vi "UDS(queue).vi"() -> ()   [LabVIEW 2020]
uses:
  <vilib>/Automotive Diagnostic Command Set/Diagnostic Transport.llb/Transport Protocol Selector.ctl
  <vilib>/Automotive Diagnostic Command Set/Diagnostic Transport.llb/Property ID.ctl
  <vilib>/addons/Automotive Diagnostic Command Set/NI_Automotive Diagnostic Command Set.lvlib
panel:
  out "Clear DTC":bool
  in  "Auto":bool
  in  "Reset":bool
  in  "Stop":bool
  in  "Option":i32(ring) items=["读软件版本", "读DTC", "清DTC"]
  in  "Action":bool
  out "open_ok?":bool
  out "Response":u8[](array[numeric]) format="%.0x"
  out "CAN_log":string[][](table)
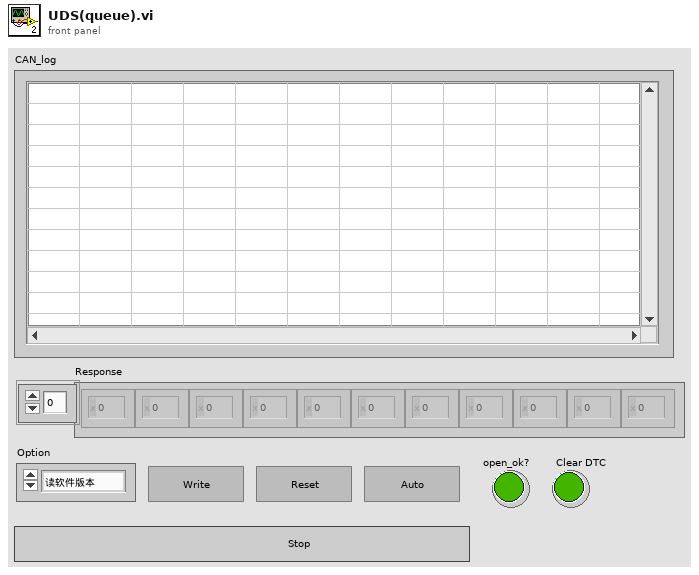
[diagram p1: front panel]
types:
  T1 = typedef "NI_Automotive Diagnostic Command Set.lvlib/Property ID.ctl" = enum16{"Timeout Diag Command", "Timeout FC (Bs)", "Timeout CF (Cr)", "Receive Block Size (BS)", "Wait Time CF (STmin)", "Max Wait Frames (N_WFTmax)", "Wait Frames to Send (N_WAIT)", "Time between Waits (T_W)", "Fill CAN Frames", "Fill Byte", "Invalid Response as Error", "Max RspPending Count", "VWTP Command Timeout", "STmin", "P2min", "Termination", "Timeout RspPending", "LIN Sleep", "Actual CAN IO Mode", "Response Plausibility Check", "Session-based Properties"}
  T2 = typedef "NI_Automotive Diagnostic Command Set.lvlib/Transport Protocol Selector.ctl" = enum16{"ISO TP - Normal Mode", "ISO TP - Mixed Mode", "VW TP 2.0", "Diagnostics on IP", "ISO TP LIN"}
  T3 = typedef "NI_Automotive Diagnostic Command Set.lvlib/Diag Reference.ctl" = cluster{"Diag CAN Handle":u32, "Transport Protocol":T2, "Receive Address Extension":u8, "Transmit Address Extension":u8, "Receive CAN Id":u32, "Transmit CAN Id":u32, "Log Frames ?":bool, "My TP Address":u8, "Other TP Address":u8, "T1":u16, "T2":u16, "T3":u16, "T4":u16, "Tx SN":u8, "Block Size":u8, "Rx SN":u8, "VW TP Initialized?":bool, "Tx block no":u8, "baud rate":u64, "Interface":string, "Channel Diag CAN Handle":u32, "UDP Connection ID":refnum<k16>, "TCP Connection ID":refnum<k5>, "Target IP Addr":u32, "Source Address":u16, "Target Address":u16, "Send Header NACK?":bool, "DLL Handle":u32, "NAD":u8, "Time Stamp read first":dbl, "Time Stamp read last":dbl, "Time Stamp write first":dbl, "Time Stamp write last":dbl, "Time Stamp write":dbl, "Time Stamp read":dbl, " I/O Mode":u32, "FD Baudrate":u64, "TX_DL":u16, "RX_DL":u16, "DoIP Protocol Version":T4, " Selected I/O Mode":u32, "TesterPresent Counter":u32, "TesterPresent Limit":u32, "TesterPresent Tick[ms]":i32, "TesterPresent RequireResponse?":bool, "TesterPresent Stored Ref?":bool, "TesterPresent Message":u8[], "TesterPresent Task Handle":i32, "TesterPresent Semaphore":T5, "Response Plausibility Check":u32, "Default Version?":bool, "Diagostic Globals":T6, "Session-based Properties?":bool}
  T4 = typedef "NI_Automotive Diagnostic Command Set.lvlib/DoIP Protocol Version.ctl" = u8
  T5 = typedef "Semaphore RefNum" = refnum<k1>
  T6 = typedef "NI_Automotive Diagnostic Command Set.lvlib/Diag Globals.ctl" = cluster{"Timeout FC (Bs)":u32, "Timeout CF (Cr)":u32, "Timeout Diag Command":u32, "Receive Block Size (BS)":u8, "Wait Time CF (STmin)":u8, "Max Waits (N_WFTmax)":u8, "Waits to Send (N_WAIT)":i32, "Time between Waits (TW)":u32, "Fill CAN Frames?":bool, "Fill Byte":u32, "Invalid Response as Error?":bool, "Max RspPending Count":u32, "VWTP Command Timeout":u32, "Transport Protocol":T2, "Diag CAN Handle":u32, "DLL Handle":u32, "Timeout RspPending":u32}
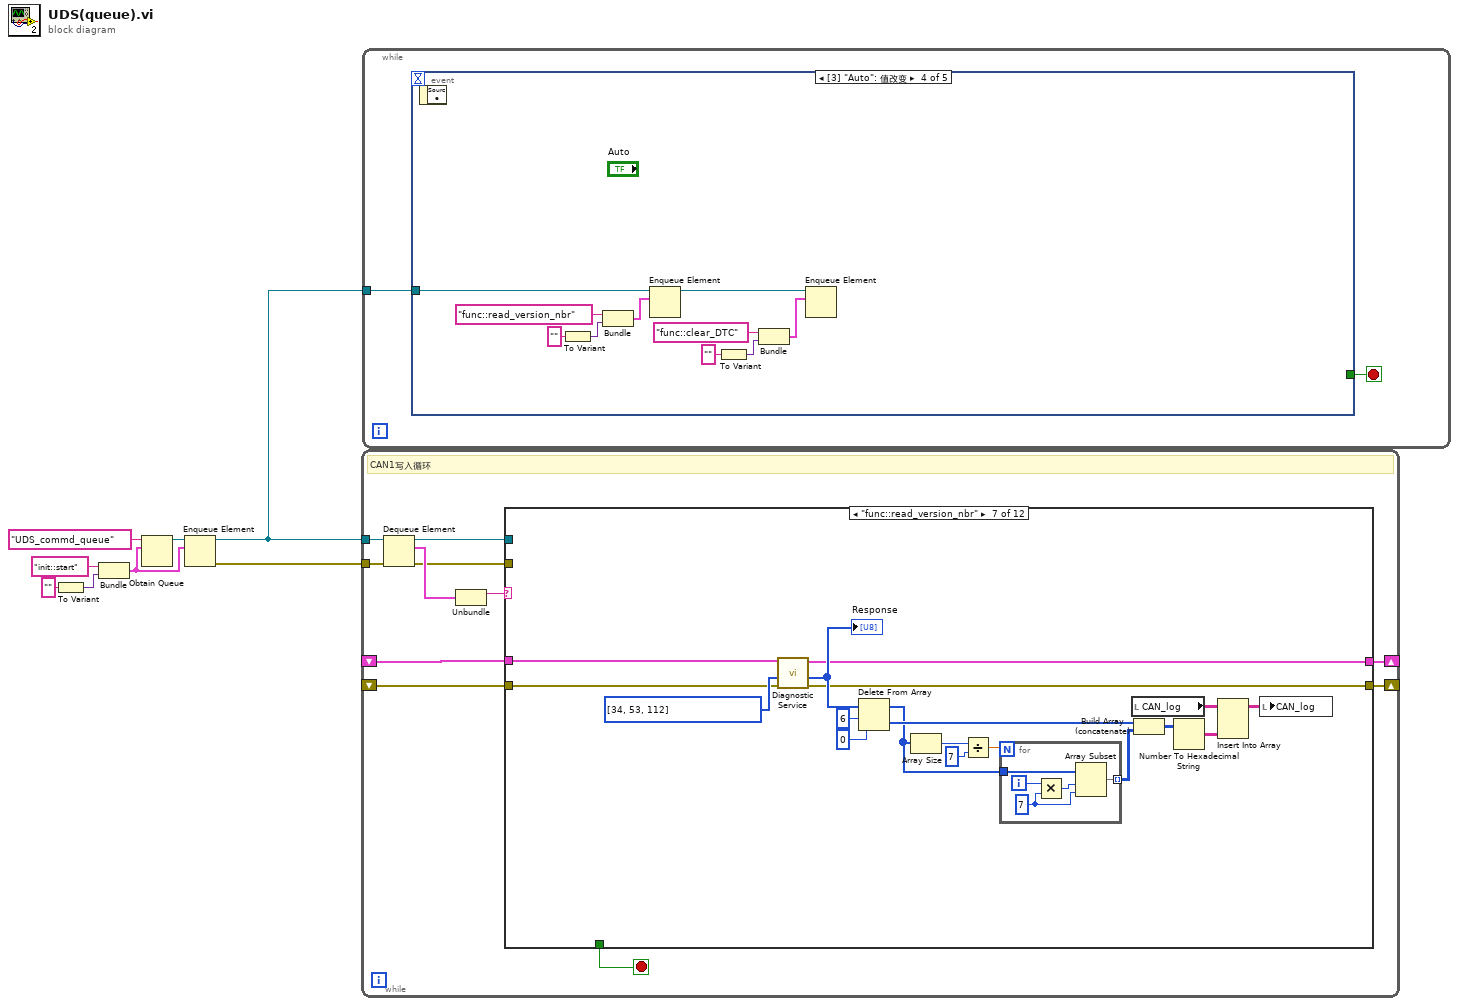
[diagram p0: block diagram]
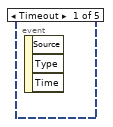
[diagram p2: hidden frame]
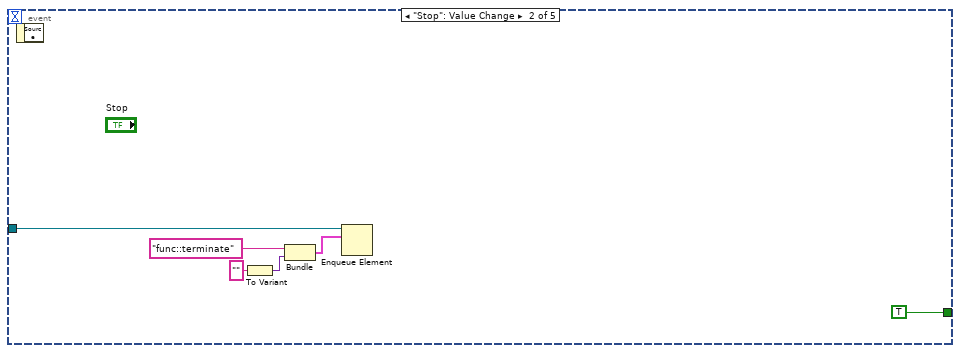
[diagram p3: hidden frame]
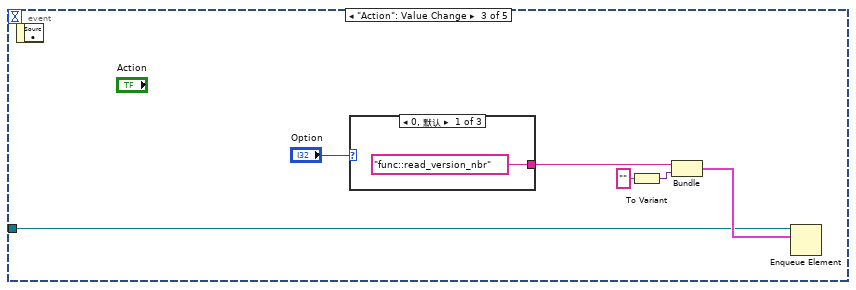
[diagram p4: hidden frame]
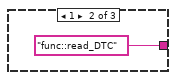
[diagram p5: hidden frame]
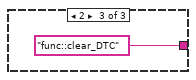
[diagram p6: hidden frame]
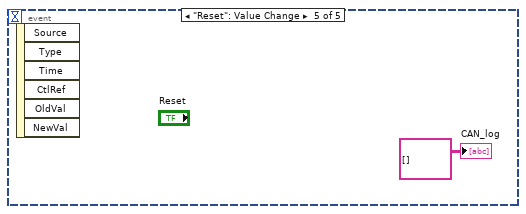
[diagram p7: hidden frame]
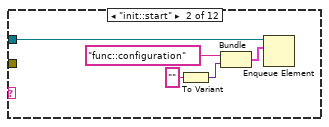
[diagram p9: hidden frame]
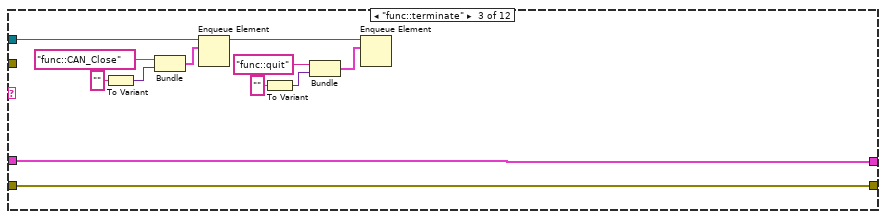
[diagram p10: hidden frame]
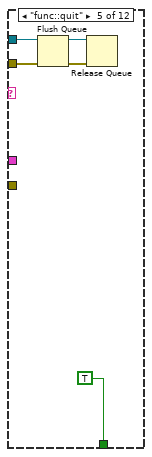
[diagram p12: hidden frame]
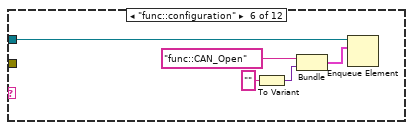
[diagram p13: hidden frame]
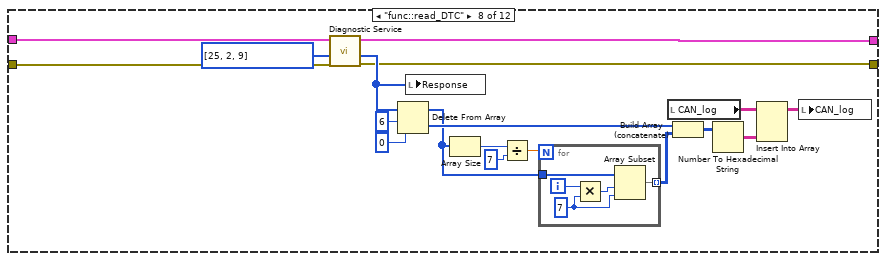
[diagram p14: hidden frame]
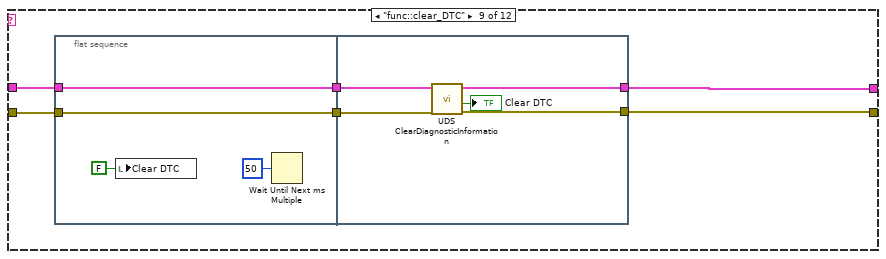
[diagram p15: hidden frame]
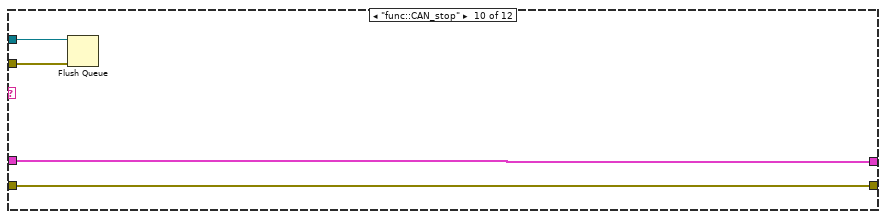
[diagram p16: hidden frame]
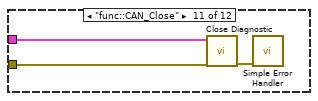
[diagram p17: hidden frame]
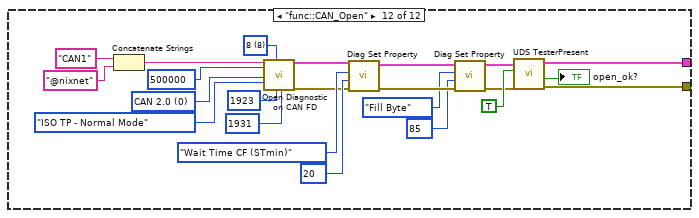
[diagram p18: hidden frame]
diagram:
  n1 = To Variant(anything="") -> (Variant=w6:variant)
  n2 = Bundle("init::start", "Variant"=w6) -> (w4:cluster{string, "Variant":variant})  [unwired: 1 in]
  n3 = Obtain Queue(name (unnamed)="UDS_commd_queue", element data type=w4) -> (queue out=w5:refnum<queue>)  [unwired: 3 in, 2 out]
  n4 = Enqueue Element(queue=w5, element=w4) -> (queue out=w2:refnum<queue>, error out=w1:errorcluster)  [unwired: 2 in, 1 out]
  n5 = while {
    tunnel: w2 -> [w18]
    tunnel: w1 -> [w15]
    shift-right: [w12] -> _
    shift-left: _ -> [w10]
    shift-right: [w11] -> _
    shift-left: _ -> [w9]
    stop <- w13 stop-if-true
    # "CAN1写入循环"
    n6 = Dequeue Element(queue=w18, error in (no error)=w15) -> (queue out=w16:refnum<queue>, element=w19:cluster{string, "Variant":variant}, error out=w14:errorcluster)  [unwired: 1 in, 1 out]
    n7 = Unbundle(w19) -> (w17:string)  [unwired: 1 out]
    n8 = case shown="\"func::read_version_nbr\"" w17 {
      tunnel: w16 -> [_ w21 w27 _ w41 w44 _ _ _ w111 _ _]
      tunnel: w14 -> [_ _ _ _ w40 _ _ _ _ w110 _ _]
      tunnel: [_ _ _ _ TRUE _ _ _ _ _ _ _] -> w13
      tunnel: [_ _ w26 w38 _ _ w50 w73 w98 w113 _ w117] -> w12
      tunnel: [_ _ w25 w37 _ _ w49 w72 w97 w112 _ w119] -> w11
      tunnel: w10 -> [_ _ w26 w38 _ _ w52 w75 w100 w113 w115 _]
      tunnel: w9 -> [_ _ w25 w37 _ _ w51 w74 w99 w112 w114 _]
      frame Default {
      }
      frame "init::start" {
        n9 = To Variant(anything="") -> (Variant=w23:variant)
        n10 = Bundle("func::configuration", "Variant"=w23) -> (w22:cluster{string, "Variant":variant})  [unwired: 1 in]
        n11 = Enqueue Element(queue=w21, element=w22) -> ()  [unwired: 2 in, 3 out]
      }
      frame "func::terminate" {
        n12 = To Variant(anything="") -> (Variant=w35:variant)
        n13 = Bundle("func::CAN_Close", "Variant"=w35) -> (w33:cluster{string, "Variant":variant})  [unwired: 1 in]
        n14 = Enqueue Element(queue=w27, element=w33) -> (queue out=w28:refnum<queue>)  [unwired: 2 in, 2 out]
        n15 = To Variant(anything="") -> (Variant=w31:variant)
        n16 = Bundle("func::quit", "Variant"=w31) -> (w29:cluster{string, "Variant":variant})  [unwired: 1 in]
        n17 = Enqueue Element(queue=w28, element=w29) -> ()  [unwired: 2 in, 3 out]
      }
      frame "func::close" {
      }
      frame "func::quit" {
        n18 = Flush Queue(queue=w41, error in (no error)=w40) -> (queue out=w43:refnum<queue>, error out=w42:errorcluster)  [unwired: 1 out]
        n19 = Release Queue(queue=w43, error in (no error)=w42) -> ()  [unwired: 1 in, 3 out]
      }
      frame "func::configuration" {
        n20 = To Variant(anything="") -> (Variant=w48:variant)
        n21 = Bundle("func::CAN_Open", "Variant"=w48) -> (w47:cluster{string, "Variant":variant})  [unwired: 1 in]
        n22 = Enqueue Element(queue=w44, element=w47) -> ()  [unwired: 2 in, 3 out]
      }
      frame "func::read_version_nbr" {
        n23 = call <vilib>:"Diagnostic Service.vi"("error in (no error)"=w51, "data in"=u8[] [34, 53, 112] ("Request"), "diag ref in"=w52) -> ("error out"=w49:errorcluster, "data out"=w57:u8[], "diag ref out"=w50:T3)  [unwired: 1 in, 5 out]
        "Response" <- w57
        n24 = Delete From Array(array=w57, length=6, index=0) -> (deleted portion=w66:u8[], array with subset deleted=w60:u8[])
        n25 = Array Size(array=w60) -> (size(s)=w58:i32)
        n26 = Divide(x=w58, y=7) -> (x/y=w59:dbl)
        n27 = for {
          N: w59 -> [_]
          tunnel: w60 -> [w71]
          tunnel: [w67] -> w61 mode=indexing
          i -> [w69]
          w70 = 7 ("length")
          n28 = Multiply(x=w69, y=w70) -> (x*y=w68:i32)
          n29 = Array Subset(array=w71, index=w68, length=w70) -> (w67:u8[])
        }
        n30 = local read "CAN_log"() -> (w62:string[][])
        n31 = Build Array (concatenate)(w66, w61) -> (w64:u8[][])
        n32 = Number To Hexadecimal String(2:w64) -> (0:w65:string[][])  [unwired: 1 in]
        n33 = Insert Into Array(array=w62, new element=w65) -> (w63:string[][])  [unwired: 2 in]
        n34 = local write "CAN_log"(w63) -> ()
      }
      frame "func::read_DTC" {
        n35 = call <vilib>:"Diagnostic Service.vi"("error in (no error)"=w74, "data in"=u8[] [25, 2, 9] ("Request"), "diag ref in"=w75) -> ("error out"=w72:errorcluster, "data out"=w79:u8[], "diag ref out"=w73:T3)  [unwired: 1 in, 5 out]
        n36 = Delete From Array(array=w79, length=6, index=0) -> (deleted portion=w83:u8[], array with subset deleted=w76:u8[])
        n37 = local write "Response"(w79) -> ()
        n38 = Array Size(array=w76) -> (size(s)=w88:i32)
        n39 = Divide(x=w88, y=7) -> (x/y=w87:dbl)
        n40 = for {
          N: w87 -> [_]
          tunnel: w76 -> [w90]
          tunnel: [w91] -> w78 mode=indexing
          i -> [w93]
          w94 = 7 ("length")
          n41 = Multiply(x=w93, y=w94) -> (x*y=w92:i32)
          n42 = Array Subset(array=w90, index=w92, length=w94) -> (w91:u8[])
        }
        n43 = local read "CAN_log"() -> (w86:string[][])
        n44 = Build Array (concatenate)(w83, w78) -> (w77:u8[][])
        n45 = Number To Hexadecimal String(2:w77) -> (0:w84:string[][])  [unwired: 1 in]
        n46 = Insert Into Array(array=w86, new element=w84) -> (w85:string[][])  [unwired: 2 in]
        n47 = local write "CAN_log"(w85) -> ()
      }
      frame "func::clear_DTC" {
        n48 = flat-sequence {
          tunnel: w99 -> [w103]
          tunnel: w100 -> [w104]
          tunnel: [w104] -> w96
          tunnel: [w103] -> w95
          tunnel: [w107] -> w98
          tunnel: [w106] -> w97
          tunnel: w96 -> [w109]
          tunnel: w95 -> [w108]
          frame #0 {
            n49 = local write "Clear DTC"(FALSE ("Clear DTC")) -> ()
            n50 = Wait Until Next ms Multiple(millisecond multiple=u32 50) -> ()  [unwired: 1 out]
          }
          frame #1 {
            n51 = call <vilib>:"UDS ClearDiagnosticInformation.vi"("error in (no error)"=w108, "diag ref in"=w109) -> ("error out"=w106:errorcluster, "success?"=→"Clear DTC":bool, "diag ref out"=w107:T3)  [unwired: 7 in]
          }
        }
      }
      frame "func::CAN_stop" {
        n52 = Flush Queue(queue=w111, error in (no error)=w110) -> ()  [unwired: 3 out]
      }
      frame "func::CAN_Close" {
        n53 = call <vilib>:"Close Diagnostic.vi"("error in (no error)"=w114, "diag ref in"=w115) -> ("error out"=w116:errorcluster)  [unwired: 9 out]
        n54 = call <vilib>:"Simple Error Handler.vi"("error in (no error)"=w116) -> ()  [unwired: 1 in, 8 out]
      }
      frame "func::CAN_Open" {
        w135 = u16 8 items=["8"=8, "12"=12, "16"=16, "20"=20, "24"=24, "32"=32, "48"=48, "64"=64] ("Max DLC")
        w137 = u32 0 items=["CAN 2.0", "CAN FD", "CAN FD+BRS", "ECU Determined"] ("IO Mode")
        n55 = Concatenate Strings("CAN1" ("Name"), "@nixnet") -> (w139:string)
        n56 = call <vilib>:"Open Diagnostic on CAN FD.vi"("CAN Interface"=w139, "Baud Rate"=u64 500000, "IO Mode"=w137, "Transport Protocol"=Transport_Protocol_Selector."ISO TP - Normal Mode", "Max DLC"=w135, "Transmit ID"=u32 1923, "Receive ID"=u32 1931) -> ("diag ref out"=w123:T3, "error out"=w121:errorcluster)  [unwired: 11 in]
        n57 = call <vilib>:"Diag Set Property.vi"("error in (no error)"=w121, "property value"=u32 20, "property ID"=Property_ID."Wait Time CF (STmin)", "diag ref in"=w123) -> ("error out"=w129:errorcluster, "diag ref out"=w128:T3)  [unwired: 6 in]
        n58 = call <vilib>:"Diag Set Property.vi"("error in (no error)"=w129, "property value"=u32 85, "property ID"=Property_ID."Fill Byte", "diag ref in"=w128) -> ("error out"=w120:errorcluster, "diag ref out"=w122:T3)  [unwired: 6 in]
        n59 = call <vilib>:"UDS TesterPresent.vi"("error in (no error)"=w120, "response required?"=TRUE, "diag ref in"=w122) -> ("error out"=w119:errorcluster, "success?"=→"open_ok?":bool, "diag ref out"=w117:T3)  [unwired: 6 out]
      }
    }
  }
  n60 = while {
    tunnel: w2 -> [w141]
    stop <- w140 stop-if-true
    n61 = event shown="[3] \"Auto\": 值改变" {
      selector: _ -> [_ _ _ _ _]
      dyn-events: _ -> [_ _ _ _ _]
      timeout: _ -> [_ _ _ _ _]
      tunnel: w141 -> [_ w144 w150 w163 _]
      tunnel: [_ TRUE _ _ _] -> w140
      event Timeout {
        n62 = event-data() -> ()  [unwired: 1 in, 3 out]
      }
      event "Stop": Value Change {
        n63 = event-data() -> ()  [unwired: 1 in, 1 out]
        n64 = To Variant(anything="") -> (Variant=w146:variant)
        n65 = Bundle("func::terminate", "Variant"=w146) -> (w143:cluster{string, "Variant":variant})  [unwired: 1 in]
        n66 = Enqueue Element(queue=w144, element=w143) -> ()  [unwired: 2 in, 3 out]
      }
      event "Action": Value Change {
        n67 = event-data() -> ()  [unwired: 1 in, 1 out]
        n68 = case shown="0, 默认" "Option" {
          tunnel: ["func::read_version_nbr" "func::read_DTC" "func::clear_DTC"] -> w148
          frame 0, Default {
          }
          frame 1 {
          }
          frame 2 {
          }
        }
        n69 = To Variant(anything="") -> (Variant=w151:variant)
        n70 = Bundle(w148, "Variant"=w151) -> (w152:cluster{string, "Variant":variant})  [unwired: 1 in]
        n71 = Enqueue Element(queue=w150, element=w152) -> ()  [unwired: 2 in, 3 out]
      }
      event "Auto": Value Change {
        n72 = event-data() -> ()  [unwired: 1 in, 1 out]
        n73 = To Variant(anything="") -> (Variant=w165:variant)
        n74 = Bundle("func::read_version_nbr", "Variant"=w165) -> (w166:cluster{string, "Variant":variant})  [unwired: 1 in]
        n75 = Enqueue Element(queue=w163, element=w166) -> (queue out=w157:refnum<queue>)  [unwired: 2 in, 2 out]
        n76 = To Variant(anything="") -> (Variant=w159:variant)
        n77 = Bundle("func::clear_DTC", "Variant"=w159) -> (w158:cluster{string, "Variant":variant})  [unwired: 1 in]
        n78 = Enqueue Element(queue=w157, element=w158) -> ()  [unwired: 2 in, 3 out]
      }
      event "Reset": Value Change {
        n79 = event-data() -> ()  [unwired: 1 in, 6 out]
        "CAN_log" <- string[][] [] ("CAN_log")
      }
    }
  }
